vi "quadratic.vi"() -> ()   [LabVIEW 2013]
panel:
  out "String":string
  out "Numeric 2":dbl
  out "Numeric":dbl
  in  "c":dbl
  in  "b":dbl
  in  "a":dbl
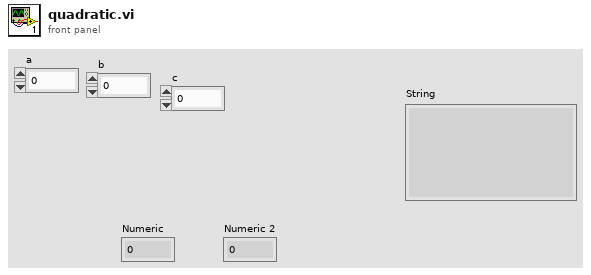
[diagram p1: front panel]
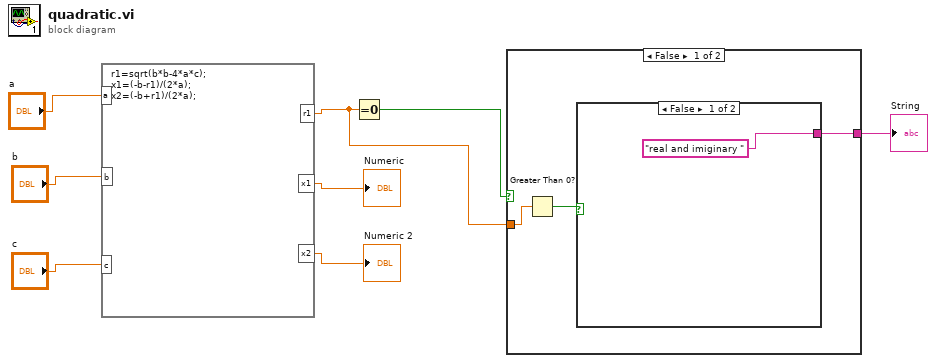
[diagram p0: block diagram]
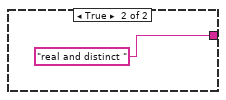
[diagram p2: hidden frame]
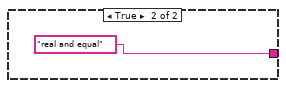
[diagram p3: hidden frame]
diagram:
  n1 = formula code="r1=sqrt(b*b-4*a*c);\nx1=(-b-r1)/(2*a);\nx2=(-b+r1)/(2*a);"("a"="a", "b"="b", "c"="c") -> ("r1"=w1:dbl, "x1"=→"Numeric":dbl, "x2"=→"Numeric 2":dbl)
  n2 = Equal To 0?(x=w1) -> (x = 0?=w3:bool)
  n3 = case shown="False" w3 {
    tunnel: [w9 "real and equal"] -> w2
    tunnel: w1 -> [w10 _]
    frame False {
      n4 = Greater Than 0?(x=w10) -> (x > 0?=w11:bool)
      n5 = case shown="False" w11 {
        tunnel: ["real and imiginary " "real and distinct "] -> w9
        frame False {
        }
        frame True {
        }
      }
    }
    frame True {
    }
  }
  "String" <- w2
